vi "PathFollower.vi"(0 "Waypoint 2":dbl[](array[numeric]), 1 "Position":dbl[](array[numeric]), 2 "Dest":dbl[](array[numeric]), 3 "Reinitialize":bool, 5 "Waypoint 1":dbl[](array[numeric]), 9 "Waypoint 0":dbl[](array[numeric]), 11 "Dest_orientation":dbl, 12 "output xy":dbl=1.0, 13 "output angle":dbl=4.0, 15 "dest_vel":dbl) -> (4 "Output\nVelocity":dbl[](array[numeric]) format="%.2f")   [LabVIEW 2018]
uses:
  <vilib>/Analysis/_algsub.llb/Real Vector Norm.vi
  <vilib>/Analysis/coordinate.llb/Wrap Angle (scalar).vi
  <vilib>/Analysis/coordinate.llb/2D Cartesian Coordinate Rotation (Scalar).vi
  <vilib>/Analysis/NI_AALPro.lvlib
  <vilib>/Analysis/NI_AAL_Angle.lvlib
panel:
  out "theta":dbl
  in  "PID gains paralelo":T1={"proportional gain (Kc)"=0.004, "integral time (Ti, min)"=0.0, "derivative time (Td, min)"=-0.07}
  out "output array":cluster{"output high":dbl, "output low":dbl}[](array[cluster])
  in  "PID Gains Angle":T1={"proportional gain (Kc)"=5.0, "integral time (Ti, min)"=0.0, "derivative time (Td, min)"=-2.0}
  in  "PID Gains lateral":T1={"proportional gain (Kc)"=0.008, "integral time (Ti, min)"=0.0, "derivative time (Td, min)"=-0.07}
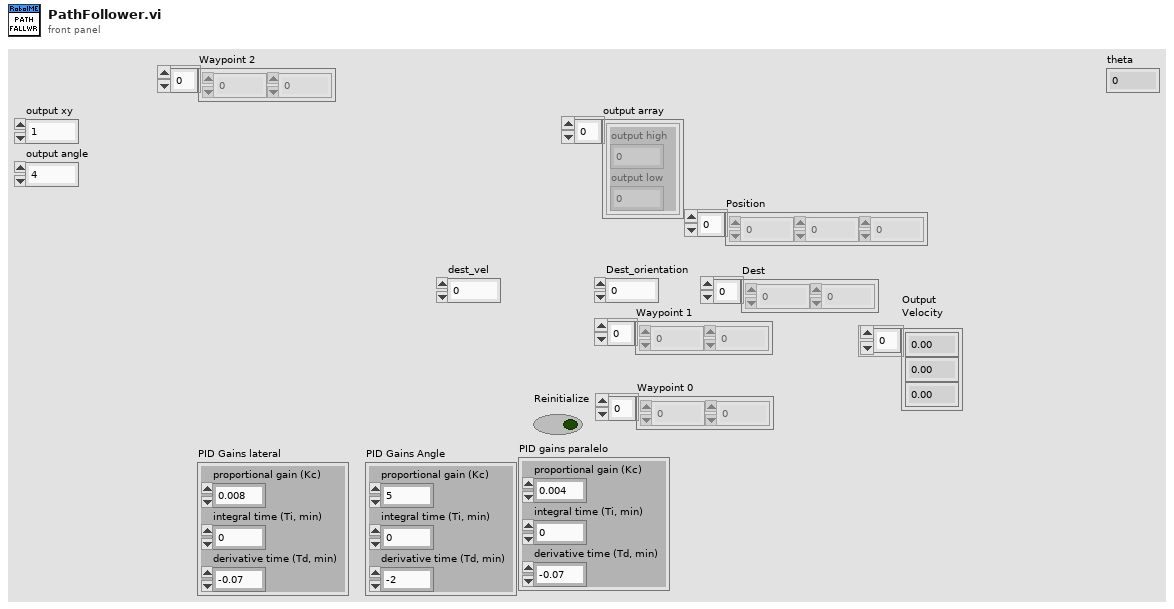
[diagram p1: front panel]
types:
  T1 = cluster{"proportional gain (Kc)":dbl, "integral time (Ti, min)":dbl, "derivative time (Td, min)":dbl}
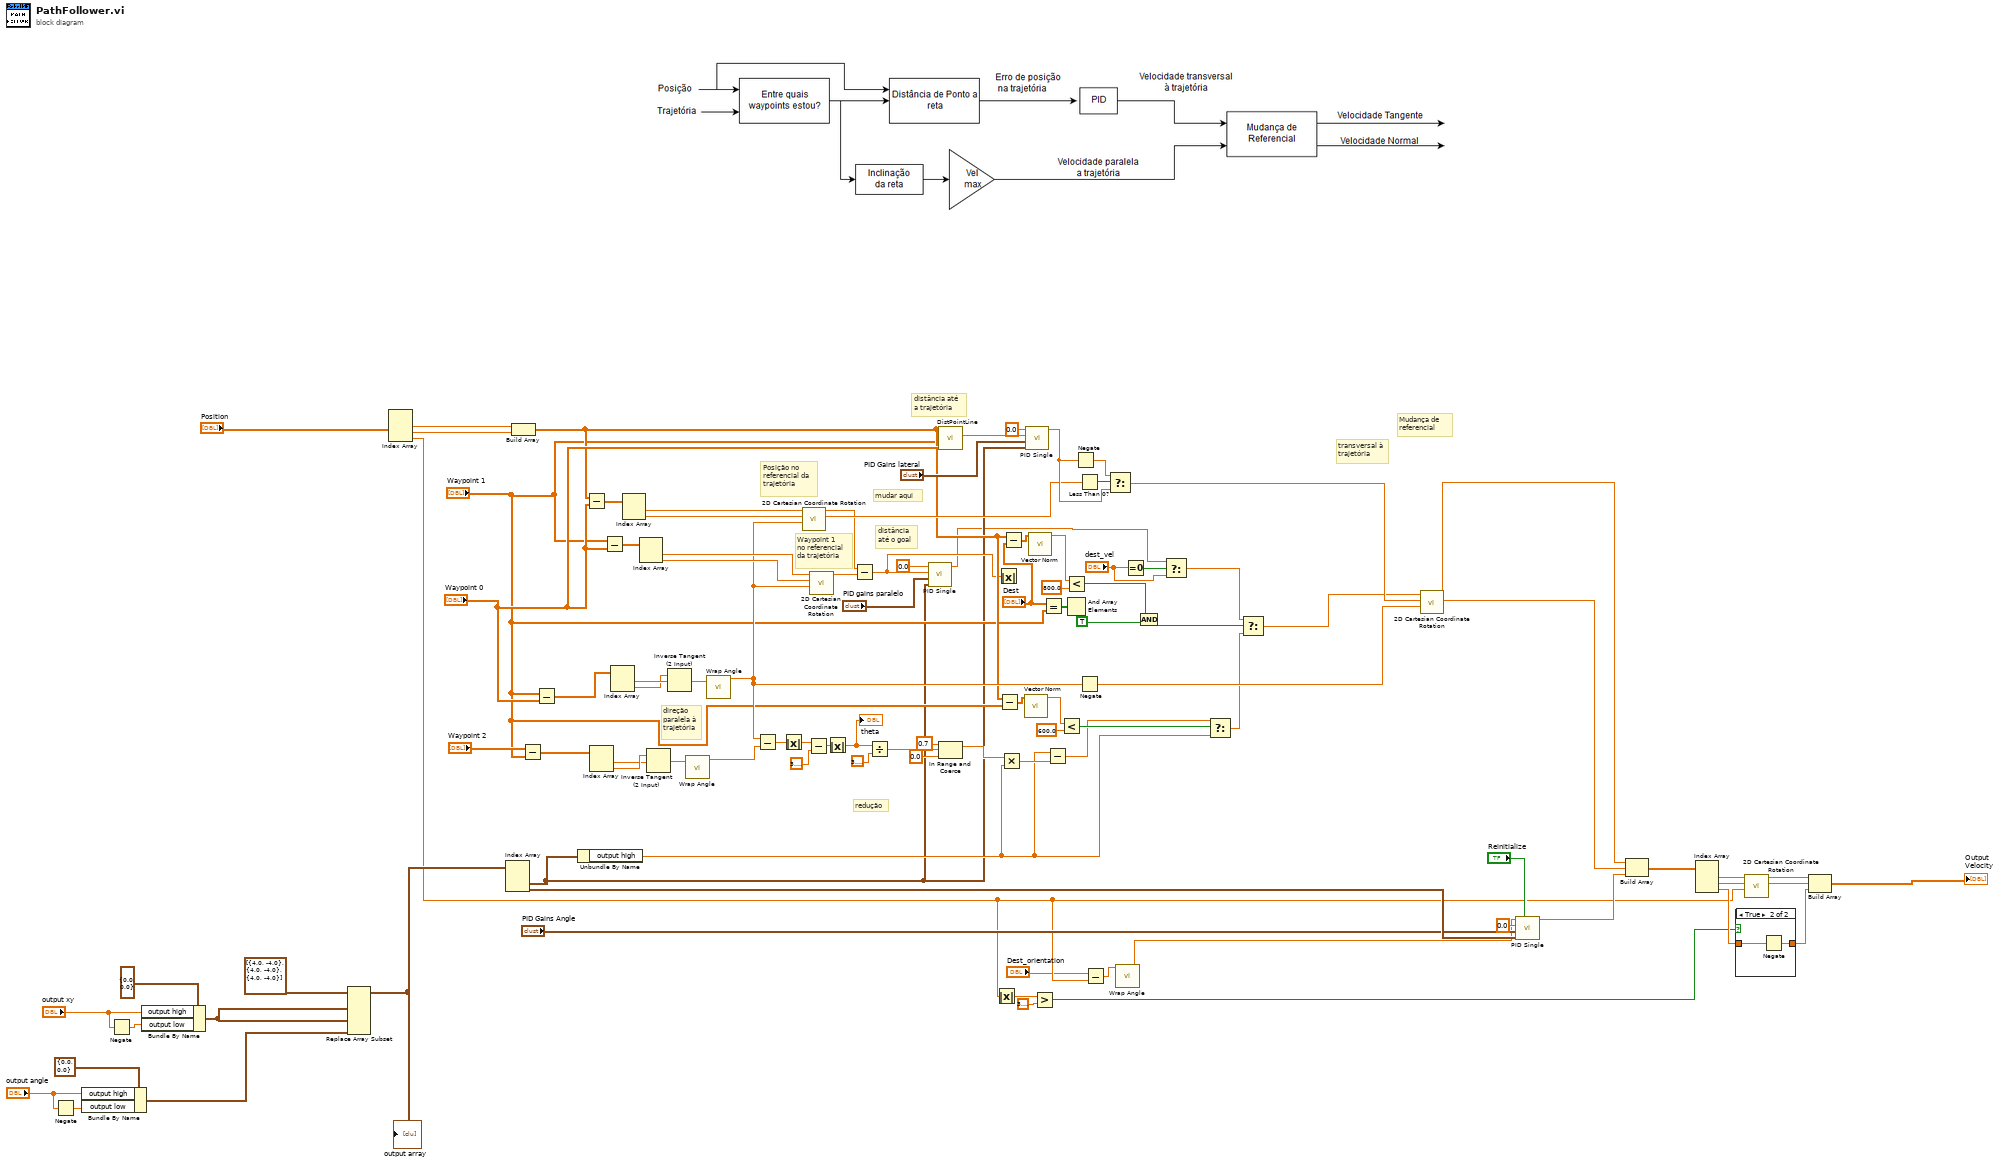
[diagram p0: block diagram]
diagram:
  # "mudar aqui"
  # "redução"
  # "Waypoint 1\nno referencial\nda trajetória"
  # "Posição no \nreferencial da\ntrajetória"
  # "distância \naté o goal"
  # "distância até \na trajetória"
  # "Mudança de \nreferencial"
  # "transversal à\ntrajetória"
  # "direção\nparalela à\ntrajetória"
  n1 = Negate(x="output angle") -> (-x=w77:dbl)
  n2 = Bundle By Name(cluster=cluster{"output high":dbl, "output low":dbl} {"output high"=0.0, "output low"=0.0}, "output high"="output angle", "output low"=w77) -> (w83:cluster{"output high":dbl, "output low":dbl})
  n3 = Negate(x="output xy") -> (-x=w79:dbl)
  n4 = Bundle By Name(cluster=cluster{"output high":dbl, "output low":dbl} {"output high"=0.0, "output low"=0.0} ("new element/subarray"), "output high"="output xy", "output low"=w79) -> (w81:cluster{"output high":dbl, "output low":dbl})
  n5 = Replace Array Subset(array=cluster{"output high":dbl, "output low":dbl}[] [{"output high"=4.0, "output low"=-4.0}, {"output high"=4.0, "output low"=-4.0}, {"output high"=4.0, "output low"=-4.0}] ("output range"), new element #1=w81, new element #2=w81, new element #3=w83) -> (w80:cluster{"output high":dbl, "output low":dbl}[])  [unwired: 3 in]
  "output array" <- w80
  n6 = Index Array(array="Position") -> (element #1=w65:dbl, element #2=w64:dbl, element #3=w74:dbl)  [unwired: 3 in]
  n7 = Index Array(array=w80) -> (element #2=w4:cluster{"output high":dbl, "output low":dbl}, element #3=w91:cluster{"output high":dbl, "output low":dbl})  [unwired: 3 in, 1 out]
  n8 = Build Array(w65, w64) -> (w22:dbl[])
  n9 = Subtract(x="Waypoint 2", y="Waypoint 1") -> (x-y=w33:dbl[])
  n10 = Subtract(x="Waypoint 1", y="Waypoint 0") -> (x-y=w52:dbl[])
  n11 = Unbundle By Name(w4) -> ("output high"=w11:dbl)
  n12 = Subtract(x=w22, y="Waypoint 0") -> (x-y=w59:dbl[])
  n13 = Index Array(array=w33) -> (element #1=w34:dbl, element #2=w36:dbl)  [unwired: 2 in]
  n14 = Subtract(x="Waypoint 1", y="Waypoint 0") -> (x-y=w50:dbl[])
  n15 = Index Array(array=w52) -> (element #1=w67:dbl, element #2=w51:dbl)  [unwired: 2 in]
  n16 = Index Array(array=w59) -> (element #1=w58:dbl, element #2=w57:dbl)  [unwired: 2 in]
  n17 = Index Array(array=w50) -> (element #1=w49:dbl, element #2=w48:dbl)  [unwired: 2 in]
  n18 = Inverse Tangent (2 Input)(1:w34, 2:w36) -> (0:w35:dbl)
  n19 = Inverse Tangent (2 Input)(1:w67, 2:w51) -> (0:w66:dbl)
  n20 = call-poly <vilib>:"Wrap Angle.vi"("angle in"=w35) -> ("angle out"=w31:dbl)  [unwired: 9 in, 1 out]
  n21 = call-poly <vilib>:"Wrap Angle.vi"("angle in"=w66) -> ("angle out"=w32:dbl)  [unwired: 9 in, 1 out]
  n22 = Subtract(x=w32, y=w31) -> (x-y=w30:dbl)
  n23 = Absolute Value(x=w30) -> (abs(x)=w29:dbl)
  n24 = call-poly <vilib>:"2D Cartesian Coordinate Rotation.vi"("theta"=w32, "y"=w57, "x"=w58) -> ("y out"=w60:dbl, "x out"=w9:dbl)  [unwired: 6 in, 1 out]
  n25 = Subtract(x=w29, y=3.141592653589793) -> (x-y=w27:dbl)
  n26 = call-poly <vilib>:"2D Cartesian Coordinate Rotation.vi"("theta"=w32, "y"=w48, "x"=w49) -> ("x out"=w8:dbl)  [unwired: 6 in, 2 out]
  n27 = Absolute Value(x=w27) -> (abs(x)=w25:dbl)
  "theta" <- w25
  n28 = Subtract(x=w9, y=w8) -> (x-y=w6:dbl)
  n29 = Divide(x=w25, y=3.141592653589793) -> (x/y=w18:dbl)
  n30 = call "PID Single.vi"("Limits"=w4, "PID gains in"="PID gains paralelo", "Variable"=w6, "Setpoint"=0.0) -> ("Out"=w3:dbl)  [unwired: 7 in]
  n31 = call "DistPointLine.vi"("P2"="Waypoint 0", "P1"="Waypoint 1", "Q"=w22) -> ("distance"=w73:dbl)  [unwired: 8 in]
  n32 = In Range and Coerce(upper limit=0.7, x=w18, lower limit=0.0) -> (coerced(x)=w15:dbl)  [unwired: 1 out]
  n33 = Absolute Value(x=w74) -> (abs(x)=w97:dbl)
  n34 = Absolute Value(x=w6) -> ()  [unwired: 1 out]
  n35 = Subtract(x=w22, y="Waypoint 1") -> (x-y=w23:dbl[])
  n36 = Multiply(x=w15, y=w11) -> (x*y=w14:dbl)
  n37 = Subtract(x=w22, y="Dest") -> (x-y=w40:dbl[])
  n38 = call-poly <vilib>:"Vector Norm.vi"("Input Vector"=w23) -> ("norm"=w19:dbl)  [unwired: 9 in, 1 out]
  n39 = call "PID Single.vi"("Limits"=w4, "PID gains in"="PID Gains lateral", "Variable"=w73, "Setpoint"=0.0) -> ("Out"=w62:dbl)  [unwired: 7 in]
  n40 = call-poly <vilib>:"Vector Norm.vi"("Input Vector"=w40) -> ("norm"=w38:dbl)  [unwired: 9 in, 1 out]
  n41 = Greater?(x=w97, y=3.141592653589793) -> (0:w92:bool)
  n42 = Equal?(x="Dest", y="Waypoint 1") -> (x = y?=w47:bool[])
  n43 = Subtract(x=w11, y=w14) -> (x-y=w12:dbl)
  n44 = Less?(x=w19, y=600.0) -> (x < y?=w13:bool)
  n45 = And Array Elements(Boolean array=w47) -> ()  [unwired: 1 out]
  n46 = Less?(x=w38, y=800.0) -> (x < y?=w44:bool)
  n47 = Negate(x=w62) -> (-x=w63:dbl)
  n48 = Less Than 0?(x=w60) -> (x < 0?=w56:bool)
  n49 = Negate(x=w32) -> (-x=w70:dbl)
  n50 = Subtract(x="Dest_orientation", y=w74) -> (x-y=w88:dbl)
  n51 = Select(t=w63, s=w56, f=w62) -> (s? t:f=w61:dbl)
  n52 = call-poly <vilib>:"Wrap Angle.vi"("angle in"=w88) -> ("angle out"=w87:dbl)  [unwired: 9 in, 1 out]
  n53 = Equal To 0?(x="dest_vel") -> (x = 0?=w43:bool)
  n54 = Compound Arithmetic op=AND(w44, TRUE ("value")) -> (w46:bool)
  n55 = Select(t=w3, s=w43, f="dest_vel") -> (s? t:f=w41:dbl)
  n56 = Select(t=w12, s=w13, f=w11) -> (s? t:f=w10:dbl)
  n57 = Select(t=w41, s=w46, f=w10) -> (s? t:f=w2:dbl)
  n58 = call-poly <vilib>:"2D Cartesian Coordinate Rotation.vi"("theta"=w70, "y"=w61, "x"=w2) -> ("y out"=w68:dbl, "x out"=w69:dbl)  [unwired: 6 in, 1 out]
  n59 = call "PID Single.vi"("initialize"="Reinitialize", "Limits"=w91, "PID gains in"="PID Gains Angle", "Variable"=0.0, "Setpoint"=w87) -> ("Out"=w93:dbl)  [unwired: 6 in]
  n60 = Build Array(w69, w68, w93) -> (w86:dbl[])
  n61 = Index Array(array=w86) -> (element #1=w101:dbl, element #2=w100:dbl, element #3=w96:dbl)  [unwired: 3 in]
  n62 = case shown="True" w92 {
    tunnel: w96 -> [w102 w104]
    tunnel: [w102 w103] -> w95
    frame False {
    }
    frame True {
      n63 = Negate(x=w104) -> (-x=w103:dbl)
    }
  }
  n64 = call-poly <vilib>:"2D Cartesian Coordinate Rotation.vi"("theta"=w74, "y"=w100, "x"=w101) -> ("y out"=w98:dbl, "x out"=w99:dbl)  [unwired: 6 in, 1 out]
  n65 = Build Array(w99, w98, w95) -> (→"Output\nVelocity":dbl[])
